vi "LoadMPCMatrix_singleAxis_variableN_80Mhz.vi"(8 "nuN_mpc":u16, 9 "Ns+1":u16, 10 "FIFO Timeout\nIn":bool) -> (0 "FIFO Matrix Timeout":bool, 3 "error out":errorcluster)   [LabVIEW 2017]
uses:
  typeDefs/QP_mem_type.ctl
  <vilib>/rvi/interface/RandomDataEmulation/niFpgaRandomDataHandleErrors.vi
  <vilib>/rvi/DataTransferAndStorage/Container/XNode/niFpgaContainer.xnode
  <vilib>/rvi/interface/RandomDataEmulation/nirviRandomDataFpgaReadWriteTemplate.vi
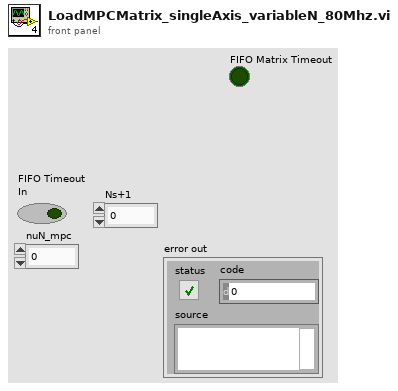
[diagram p1: front panel]
types:
  T1 = typedef "QP_mem_type.ctl" = refnum<k21>
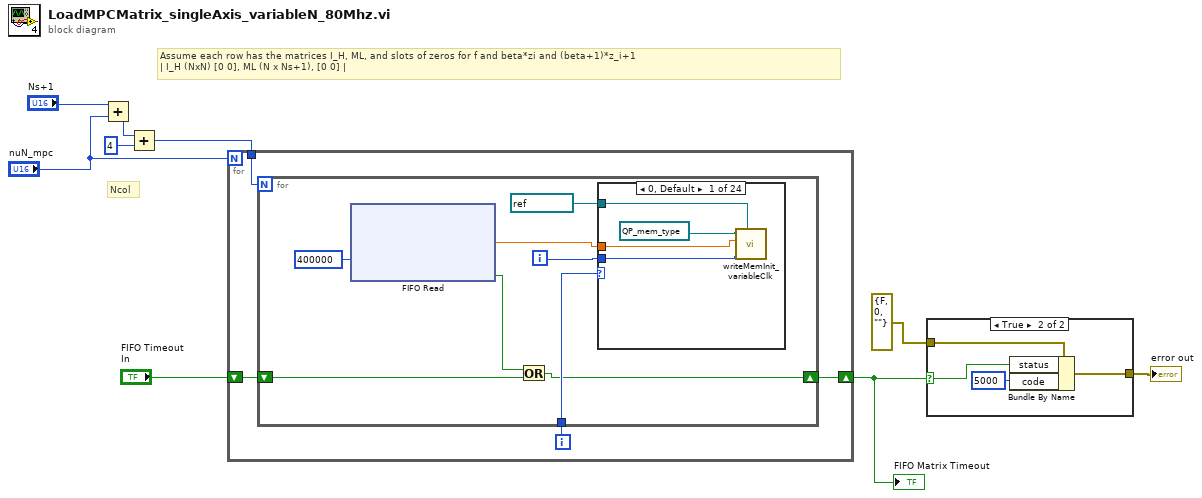
[diagram p0: block diagram]
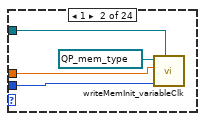
[diagram p2: hidden frame]
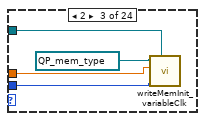
[diagram p3: hidden frame]
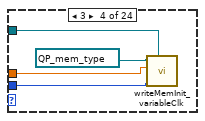
[diagram p4: hidden frame]
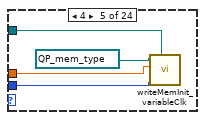
[diagram p5: hidden frame]
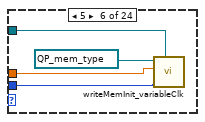
[diagram p6: hidden frame]
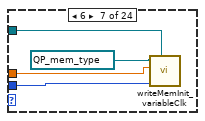
[diagram p7: hidden frame]
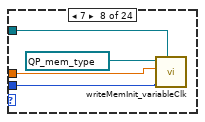
[diagram p8: hidden frame]
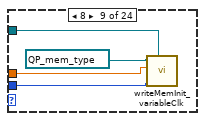
[diagram p9: hidden frame]
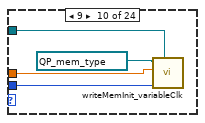
[diagram p10: hidden frame]
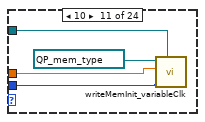
[diagram p11: hidden frame]
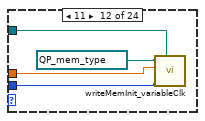
[diagram p12: hidden frame]
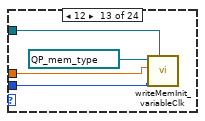
[diagram p13: hidden frame]
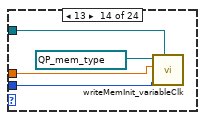
[diagram p14: hidden frame]
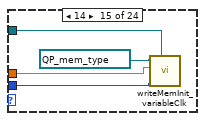
[diagram p15: hidden frame]
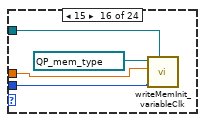
[diagram p16: hidden frame]
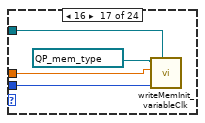
[diagram p17: hidden frame]
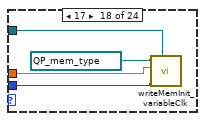
[diagram p18: hidden frame]
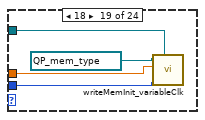
[diagram p19: hidden frame]
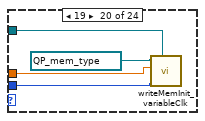
[diagram p20: hidden frame]
diagram:
  # "Ncol"
  # "Assume each row has the matrices I_H, ML, and slots of zeros for f and beta*zi and (beta+1)*z_i+1\n| I_H (NxN) [0 0], ML (N x Ns+1), [0 0] |"
  n1 = Add(x="Ns+1", y="nuN_mpc") -> (x+y=w7:u16)
  n2 = Add(x=w7, y=u16 4) -> (x+y=w5:u16)
  n3 = for {
    N: "nuN_mpc" -> [_]
    tunnel: w5 -> [w13]
    shift-right: [w10] -> w3
    shift-left: "FIFO Timeout\nIn" -> [w11]
    i -> [w12]
    n4 = for {
      N: w13 -> [_]
      tunnel: w12 -> [w18]
      shift-right: [w15] -> w10
      shift-left: w11 -> [w16]
      i -> [w20]
      n5 = xnode ("FIFO Read")("Timeout"=400000) -> ("Element"=w19:sgl, "Timed Out?"=w17:bool)  [unwired: 1 in, 1 out]
      n6 = Or(x=w17, y=w16) -> (x .or. y?=w15:bool)
      n7 = case shown="0, Default" w18 {
        tunnel: w19 -> [w23 w26 w31 w36 w40 w43 w48 w52 w56 w60 w64 w68 w72 w76 w80 w83 w88 w92 w96 w99 w104 w108 w112 w116]
        tunnel: w20 -> [w24 w27 w30 w35 w39 w42 w47 w51 w55 w59 w63 w67 w71 w75 w79 w84 w87 w91 w95 w98 w103 w106 w110 w114]
        tunnel: refnum<k21> "80MHz" ("Clk") -> [w22 w28 w32 w34 w38 w44 w46 w50 w54 w58 w62 w66 w70 w74 w78 w82 w86 w90 w94 w100 w102 w107 w111 w115]
        frame 0, Default {
          n8 = call "writeMemInit_variableClk.vi"("Clk"=w22, "address"=w24, "data"=w23, "QP-Memory In"=T1 "Memory" ("Memory In")) -> ()  [unwired: 8 in]
        }
        frame 1 {
          n9 = call "writeMemInit_variableClk.vi"("Clk"=w28, "address"=w27, "data"=w26, "QP-Memory In"=T1 "Memory 2" ("Memory In")) -> ()  [unwired: 8 in]
        }
        frame 2 {
          n10 = call "writeMemInit_variableClk.vi"("Clk"=w32, "address"=w30, "data"=w31, "QP-Memory In"=T1 "Memory 3" ("Memory In")) -> ()  [unwired: 8 in]
        }
        frame 3 {
          n11 = call "writeMemInit_variableClk.vi"("Clk"=w34, "address"=w35, "data"=w36, "QP-Memory In"=T1 "Memory 4" ("Memory In")) -> ()  [unwired: 8 in]
        }
        frame 4 {
          n12 = call "writeMemInit_variableClk.vi"("Clk"=w38, "address"=w39, "data"=w40, "QP-Memory In"=T1 "Memory 5" ("Memory In")) -> ()  [unwired: 8 in]
        }
        frame 5 {
          n13 = call "writeMemInit_variableClk.vi"("Clk"=w44, "address"=w42, "data"=w43, "QP-Memory In"=T1 "Memory 6" ("Memory In")) -> ()  [unwired: 8 in]
        }
        frame 6 {
          n14 = call "writeMemInit_variableClk.vi"("Clk"=w46, "address"=w47, "data"=w48, "QP-Memory In"=T1 "Memory 7" ("Memory In")) -> ()  [unwired: 8 in]
        }
        frame 7 {
          n15 = call "writeMemInit_variableClk.vi"("Clk"=w50, "address"=w51, "data"=w52, "QP-Memory In"=T1 "Memory 8" ("Memory In")) -> ()  [unwired: 8 in]
        }
        frame 8 {
          n16 = call "writeMemInit_variableClk.vi"("Clk"=w54, "address"=w55, "data"=w56, "QP-Memory In"=T1 "Memory 9" ("Memory In")) -> ()  [unwired: 8 in]
        }
        frame 9 {
          n17 = call "writeMemInit_variableClk.vi"("Clk"=w58, "address"=w59, "data"=w60, "QP-Memory In"=T1 "Memory 10" ("Memory In")) -> ()  [unwired: 8 in]
        }
        frame 10 {
          n18 = call "writeMemInit_variableClk.vi"("Clk"=w62, "address"=w63, "data"=w64, "QP-Memory In"=T1 "Memory 11" ("Memory In")) -> ()  [unwired: 8 in]
        }
        frame 11 {
          n19 = call "writeMemInit_variableClk.vi"("Clk"=w66, "address"=w67, "data"=w68, "QP-Memory In"=T1 "Memory 12" ("Memory In")) -> ()  [unwired: 8 in]
        }
        frame 12 {
          n20 = call "writeMemInit_variableClk.vi"("Clk"=w70, "address"=w71, "data"=w72, "QP-Memory In"=T1 "Memory 13" ("Memory In")) -> ()  [unwired: 8 in]
        }
        frame 13 {
          n21 = call "writeMemInit_variableClk.vi"("Clk"=w74, "address"=w75, "data"=w76, "QP-Memory In"=T1 "Memory 14" ("Memory In")) -> ()  [unwired: 8 in]
        }
        frame 14 {
          n22 = call "writeMemInit_variableClk.vi"("Clk"=w78, "address"=w79, "data"=w80, "QP-Memory In"=T1 "Memory 15" ("Memory In")) -> ()  [unwired: 8 in]
        }
        frame 15 {
          n23 = call "writeMemInit_variableClk.vi"("Clk"=w82, "address"=w84, "data"=w83, "QP-Memory In"=T1 "Memory 16" ("Memory In")) -> ()  [unwired: 8 in]
        }
        frame 16 {
          n24 = call "writeMemInit_variableClk.vi"("Clk"=w86, "address"=w87, "data"=w88, "QP-Memory In"=T1 "Memory 17" ("Memory In")) -> ()  [unwired: 8 in]
        }
        frame 17 {
          n25 = call "writeMemInit_variableClk.vi"("Clk"=w90, "address"=w91, "data"=w92, "QP-Memory In"=T1 "Memory 18" ("Memory In")) -> ()  [unwired: 8 in]
        }
        frame 18 {
          n26 = call "writeMemInit_variableClk.vi"("Clk"=w94, "address"=w95, "data"=w96, "QP-Memory In"=T1 "Memory 19" ("Memory In")) -> ()  [unwired: 8 in]
        }
        frame 19 {
          n27 = call "writeMemInit_variableClk.vi"("Clk"=w100, "address"=w98, "data"=w99, "QP-Memory In"=T1 "Memory 20" ("Memory In")) -> ()  [unwired: 8 in]
        }
        frame 20 {
          n28 = call "writeMemInit_variableClk.vi"("Clk"=w102, "address"=w103, "data"=w104, "QP-Memory In"=T1 "Memory 21" ("Memory In")) -> ()  [unwired: 8 in]
        }
        frame 21 {
          n29 = call "writeMemInit_variableClk.vi"("Clk"=w107, "address"=w106, "data"=w108, "QP-Memory In"=T1 "Memory 22" ("Memory In")) -> ()  [unwired: 8 in]
        }
        frame 22 {
          n30 = call "writeMemInit_variableClk.vi"("Clk"=w111, "address"=w110, "data"=w112, "QP-Memory In"=T1 "Memory 23" ("Memory In")) -> ()  [unwired: 8 in]
        }
        frame 23 {
          n31 = call "writeMemInit_variableClk.vi"("Clk"=w115, "address"=w114, "data"=w116, "QP-Memory In"=T1 "Memory 24" ("Memory In")) -> ()  [unwired: 8 in]
        }
      }
    }
  }
  "FIFO Matrix Timeout" <- w3
  n32 = case shown="True" w3 {
    selector: w3 -> [_ w121]
    tunnel: errorcluster {"status"=FALSE, "code"=0, "source"=""} ("error in") -> [w118 w122]
    tunnel: [w118 w120] -> w9
    frame False {
    }
    frame True {
      n33 = Bundle By Name(cluster=w122, "status"=w121, "code"=5000) -> (w120:errorcluster)
    }
  }
  "error out" <- w9
